vi "Build Parameters.vi"() -> (2 "Scenarios out":T1(array[cluster]))   [LabVIEW 2020, in "test.lvlib" / "01_ImageFileIO.lvclass"]
doc: "This helper function simplifies the syntax of creating parameters."
uses:
  01_ImageFileIO.lvclass
  01_ImageFileIO.lvclass/01_ImageFileIO.ctl
  Types.ctl
  8415d65c-3b73-44f2-acb5-dcc8c6bcf86c.vi
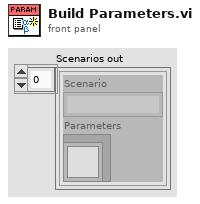
[diagram p1: front panel]
types:
  T1 = cluster{"Scenario":string, "Parameters":refnum<class "01_ImageFileIO.lvclass">}[]
  T2 = typedef "test.lvlib/01_ImageFileIO.lvclass/Types.ctl" = enum16{"jpeg", "png", "webp", "tiff"}
  T3 = cluster{string, "Parameters":refnum<class "01_ImageFileIO.lvclass">}
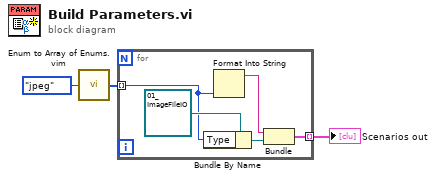
[diagram p0: block diagram]
diagram:
  n1 = call "Enum to Array of Enums.vim"("enum"=Types."jpeg" ("Types")) -> ("array of enums"=w2:T2[])
  n2 = for {
    tunnel: [w6] -> w1 mode=indexing
    tunnel: w2 -> [w5] mode=indexing
    n3 = Bundle By Name(cluster=refnum<class "01_ImageFileIO.lvclass"> refnum ("Parameters"), "Type"=w5) -> (w7:refnum<class "01_ImageFileIO.lvclass">)
    n4 = Format Into String(w5) -> (resulting string=w4:string)  [unwired: 3 in, 1 out]
    n5 = Bundle(w4, "Parameters"=w7) -> (w6:T3)  [unwired: 1 in]
  }
  "Scenarios out" <- w1
